vi "题目四.vi"() -> ()   [LabVIEW 2017]
uses:
  <vilib>/Analysis/2dsp.llb/Real FFT.vi
  <vilib>/Analysis/NI_AALPro.lvlib
  <vilib>/measure/NI_MABase.lvlib
panel:
  in  "sampling info":cluster{"Fs":dbl, "#s":dbl}={"Fs"=1000.0, "#s"=1000.0} caption="采样信息" {"Fs" format="%.2p"}
  out "时域信号 2":dbl[](graph)
  out "频域信号 2":dbl[](graph)
  in  "幅值 3":dbl=1.0 caption="幅值3" format="%0.2p"
  in  "频率3":dbl=10.0 format="%0.2p"
  in  "幅值 2":dbl=1.0 caption="幅值2" format="%0.2p"
  in  "频率 2":dbl=10.0 caption="频率2" format="%0.2p"
  in  "幅值1":dbl=1.0 format="%0.2p"
  in  "频率1":dbl=10.0 format="%0.2p"
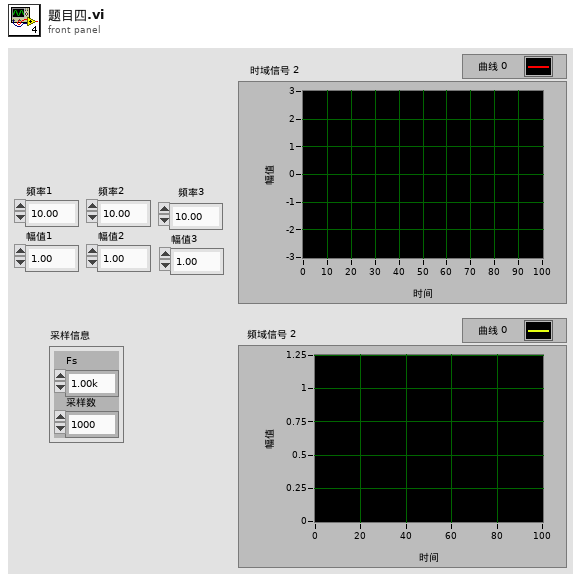
[diagram p1: front panel]
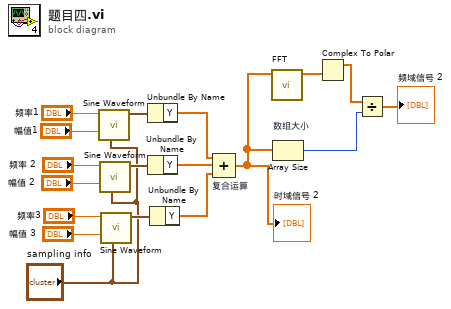
[diagram p0: block diagram]
diagram:
  n1 = call <vilib>:"Sine Waveform.vi"("sampling info"="sampling info", "amplitude"="幅值1", "frequency"="频率1") -> ("signal out"=w7:waveform(dbl))  [unwired: 7 in, 1 out]
  n2 = call <vilib>:"Sine Waveform.vi"("sampling info"="sampling info", "amplitude"="幅值 2", "frequency"="频率 2") -> ("signal out"=w6:waveform(dbl))  [unwired: 7 in, 1 out]
  n3 = call <vilib>:"Sine Waveform.vi"("sampling info"="sampling info", "amplitude"="幅值 3", "frequency"="频率3") -> ("signal out"=w5:waveform(dbl))  [unwired: 7 in, 1 out]
  n4 = Unbundle By Name(w7) -> ("Y"=w4:dbl[])
  n5 = Unbundle By Name(w6) -> ("Y"=w3:dbl[])
  n6 = Unbundle By Name(w5) -> ("Y"=w2:dbl[])
  n7 = Compound Arithmetic op=ADD "复合运算"(w4, w3, w2) -> (w8:dbl[])
  "时域信号 2" <- w8
  n8 = call-poly <vilib>:"FFT.vi"("X"=w8) -> ("FFT {X}"=w12:cdb[])  [unwired: 9 in, 1 out]
  n9 = Array Size "数组大小"(array=w8) -> (size(s)=w10:i32)
  n10 = Complex To Polar(r * e^(i*theta)=w12) -> (r=w11:dbl[])  [unwired: 1 out]
  n11 = Divide(x=w11, y=w10) -> (x/y=→"频域信号 2":dbl[])
